vi "Get Cluster Names.vi"(8 "error in":errorcluster, 11 "Test Information":T1) -> (0 "error out":errorcluster, 3 "Cluster Names":string[](array[string]))   [LabVIEW 2018, in "File IO.lvlib"]
doc: "Take the cluster reference and obtain an array of the cluster string names."
uses:
  File IO.lvlib
  Controller (Host)/Public Controls/Test Information.ctl
  Controller (Host)/Controller (Host).lvlib
panel:
  # "Test Information:"
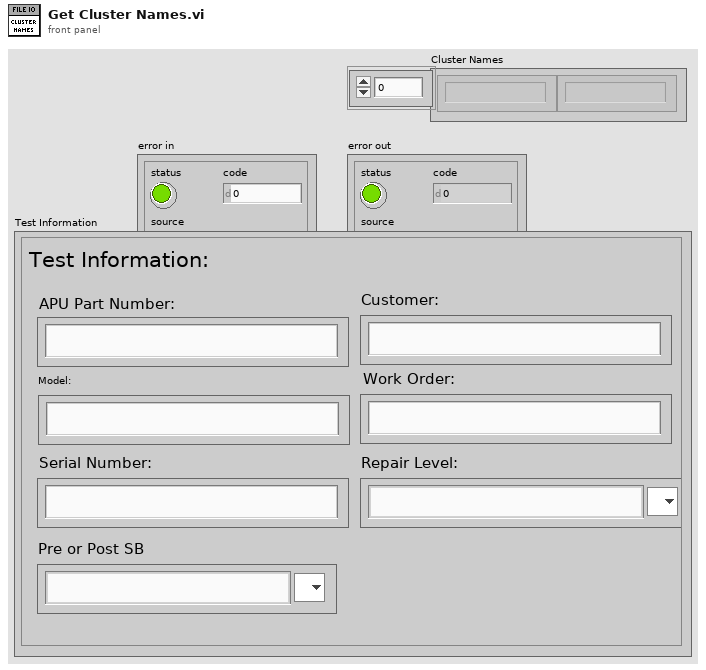
[diagram p1: front panel]
types:
  T1 = typedef "Controller (Host).lvlib/Test Information.ctl" = cluster{"APU Part Number:":string, "Model:":string, "Serial Number:":string, "Customer:":string, "Work Order:":string, "Repair Level:":string, "Pre or Post SB":string}
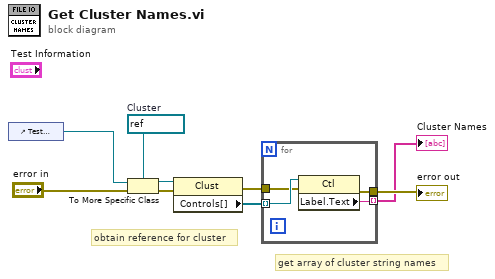
[diagram p0: block diagram]
diagram:
  w2 = refnum<vi> refnum  # Cluster
  # "get array of cluster string names"
  # "obtain reference for cluster"
  n1 = control-ref of="Test Information"() -> (w1:refnum<vi>)
  n2 = To More Specific Class(target class=w2, reference=w1, error in="error in") -> (specific class reference=w3:refnum<vi>, error out=w4:errorcluster)
  n3 = property class="Clust"(reference=w3, error in=w4) -> (error out=w6:errorcluster, "Controls[]"=w5:refnum<vi>[])  [unwired: 1 out]
  n4 = for {
    tunnel: w5 -> [w13] mode=indexing
    tunnel: w6 -> [w12]
    tunnel: [w11] -> w7 mode=indexing
    tunnel: [w10] -> w9
    n5 = property class="Ctl"(reference=w13, error in=w12) -> (error out=w10:errorcluster, "Label.Text"=w11:string)  [unwired: 1 out]
  }
  "error out" <- w9
  "Cluster Names" <- w7
